vi "Hello-C.vi"(11 "Params":string[][](array[string])) -> ()   [LabVIEW 2017]
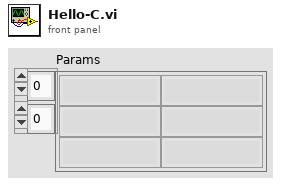
[diagram p1: front panel]
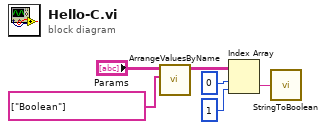
[diagram p0: block diagram]
diagram:
  n1 = call "ArrangeValuesByName.vi"("Names"=string[] ["Boolean"], "Names/Values in"="Params") -> ("Names/Values Out"=w4:string[][])  [unwired: 9 in]
  n2 = Index Array(array=w4, index (row)=0, index (col)=1) -> (element=w1:string)
  n3 = call "StringToBoolean.vi"("String"=w1) -> ()  [unwired: 1 out]
